vi "start listwave.vi"(6 "offset":u16, 7 "length":u16, 8 "error in (no error)":errorcluster, 9 "dec_ratio":u16, 10 "time":dbl, 11 "identifier":string) -> (0 "error out":errorcluster, 3 "function return":u32)   [LabVIEW 2015, in "XGL_DPP.lvlib"]
doc: "EXTERN DECLSPEC uint32_t CALL_CONV start_listwave(const char * identifier, const double time, uint16_t dec_ratio, uint16_t length, uint16_t offset);"
uses:
  XGL_DPP.lvlib
  XGL_DPP.dll
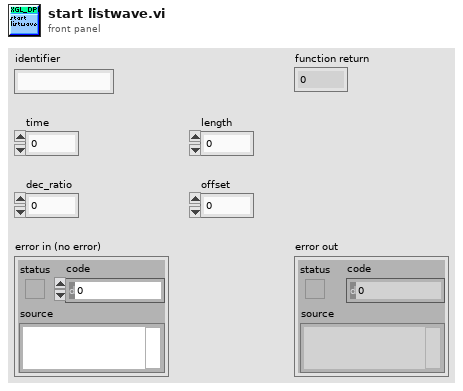
[diagram p1: front panel]
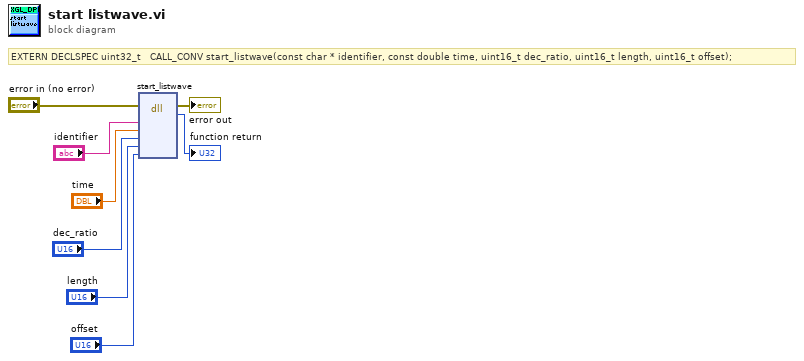
[diagram p0: block diagram]
diagram:
  # "EXTERN DECLSPEC uint32_t   CALL_CONV start_listwave(const char * identifier, const double time, uint16_t dec_ratio, uint16_t length, uint16_t offset);"
  n1 = dll-call lib="D:/Users/XRF/Desktop/Scanning Software_Demokritos_2015_v7/libs/Vis_2/XGL_DPP.*" fn="start_listwave"(error in="error in (no error)", "identifier"="identifier", "time"="time", "dec_ratio"="dec_ratio", "length"="length", "offset"="offset") -> (error out=→"error out":errorcluster, →"function return":u32)  [unwired: 7 in, 1 out]
